vi "Get Path Regex.vi"(8 "error in (no error)":errorcluster, 11 "User API in":refnum<class "User API.lvclass">) -> (0 "error out":errorcluster, 2 "Path Regex":string, 3 "User API out":refnum<class "User API.lvclass">)   [LabVIEW 2020, in "Summer of LabVIEW.lvlib" / "User API.lvclass"]
uses:
  User API.lvclass
  User API.lvclass/User API.ctl
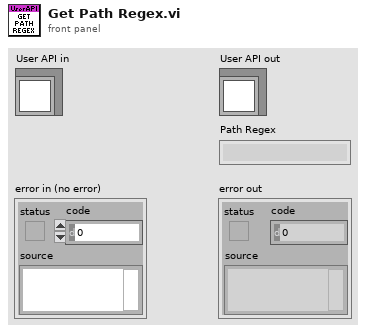
[diagram p1: front panel]
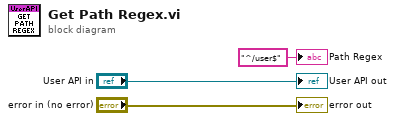
[diagram p0: block diagram]
diagram:
  "error out" <- "error in (no error)"
  "User API out" <- "User API in"
  "Path Regex" <- "^/user$" ("Path Regex")
